vi "Move Aberration Correction Lens.vi"(0 "VISA Resource Name":refnum<visa-resource-name>, 5 "Device Number (1)":i32=1, 7 "Direction (0: Opposite)":enum16{"Opposite", "Toward"}(ring), 9 "Step (0)":i32, 11 "error in (no error)":errorcluster {"code" format="%.0x"}) -> (4 "VISA Resource Name Out":refnum<visa-resource-name>, 15 "error out":errorcluster {"code" format="%.0x"})   [LabVIEW 2018, in "Olympus IX BX Series.lvlib"]
doc: "Moves the aberration correction lens.\n\nNotes:\n(1) The aberration correction lens is moved to a relative address (in the distance from the current position).\n(2) This VI is valid only for Active Autp Focus Control Unit (A1M)."
uses:
  Olympus IX BX Series.lvlib
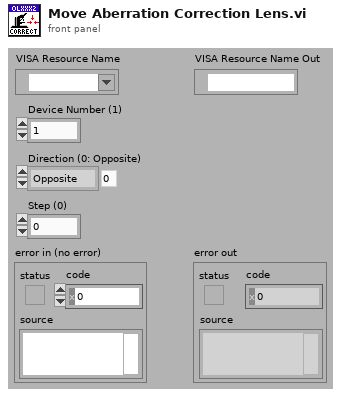
[diagram p1: front panel]
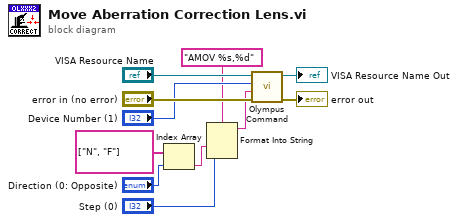
[diagram p0: block diagram]
diagram:
  n1 = Index Array(array=string[] ["N", "F"], index="Direction (0: Opposite)") -> (element=w9:string)
  n2 = Format Into String(format string="AMOV %s,%d", w9, "Step (0)") -> (resulting string=w4:string)  [unwired: 2 in, 1 out]
  n3 = call "Olympus Command.vi"("error in (no error)"="error in (no error)", "Command string"=w4, "Device Number (1)"="Device Number (1)", "VISA Resource Name"="VISA Resource Name") -> ("error out"=→"error out":errorcluster, "VISA Resource Name Out"=→"VISA Resource Name Out":refnum<visa-resource-name>)  [unwired: 5 in, 1 out]
